vi "global_sound_task_id.vi"() -> ()   [LabVIEW 2011]
uses:
  <vilib>/sound2/lvsound2.llb/Sound Output Task ID.ctl
panel:
  in  "task ID":T1 format="%.0x"
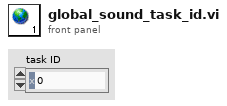
[diagram p1: front panel]
types:
  T1 = typedef "Sound Output Task ID.ctl" = u32
diagram:
